vi "Read Configuration Name.vi"(8 "error in":errorcluster, 11 "PL_System Configuration in":refnum<class "PL_System Configuration.lvclass">) -> (0 "error out":errorcluster, 2 "Configuration Name":string, 3 "PL_System Configuration out":refnum<class "PL_System Configuration.lvclass">)   [LabVIEW 2013, in "PL_System Configuration.lvclass"]
uses:
  PL_System Configuration.lvclass
  PL_System Configuration.lvclass/PL_System Configuration.ctl
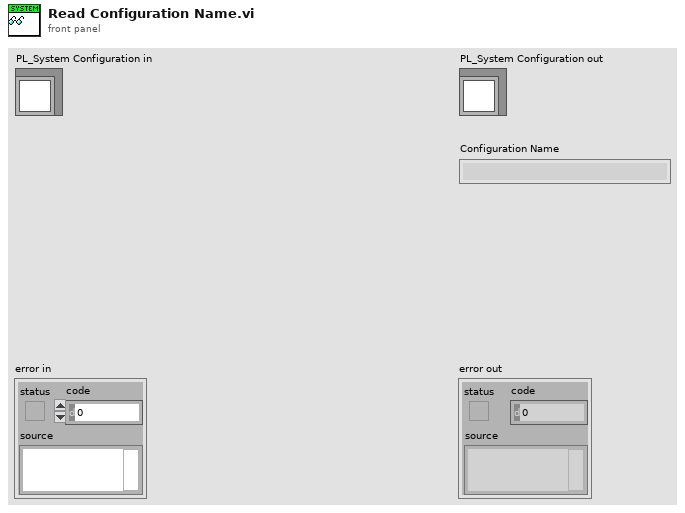
[diagram p1: front panel]
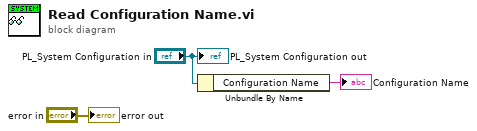
[diagram p0: block diagram]
diagram:
  n1 = Unbundle By Name("PL_System Configuration in") -> ("Configuration Name"=→"Configuration Name":string)
  "error out" <- "error in"
  "PL_System Configuration out" <- "PL_System Configuration in"
